vi "test timestamp from be bytes.vi"(8 "error in (no error)":errorcluster, 11 "TestCase in":refnum<class "Timestamp Tests.lvclass">) -> (0 "error out":errorcluster, 3 "TestCase out":refnum<class "Timestamp Tests.lvclass">)   [LabVIEW 2020, in "Timestamp Tests.lvclass"]
uses:
  Timestamp Tests.lvclass
  <vilib>/Utility/file.llb/Application Directory.vi
  <vilib>/Utility/libraryn.llb/Check if File or Folder Exists.vi
  <vilib>/addons/_JKI Toolkits/VI Tester/TestCase.llb/TestCase.lvclass
  C:/Program Files/National Instruments/LabVIEW 2024/vi.lib/addons/_JKI Toolkits/VI Tester/TestCase.llb/TestCase.lvclass
panel:
  out "data string":string
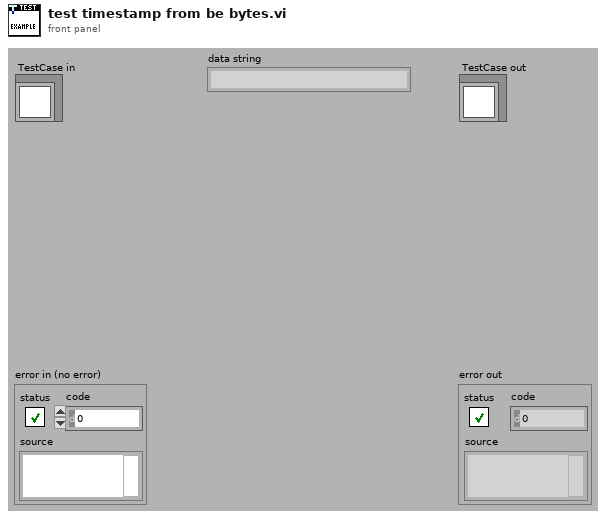
[diagram p1: front panel]
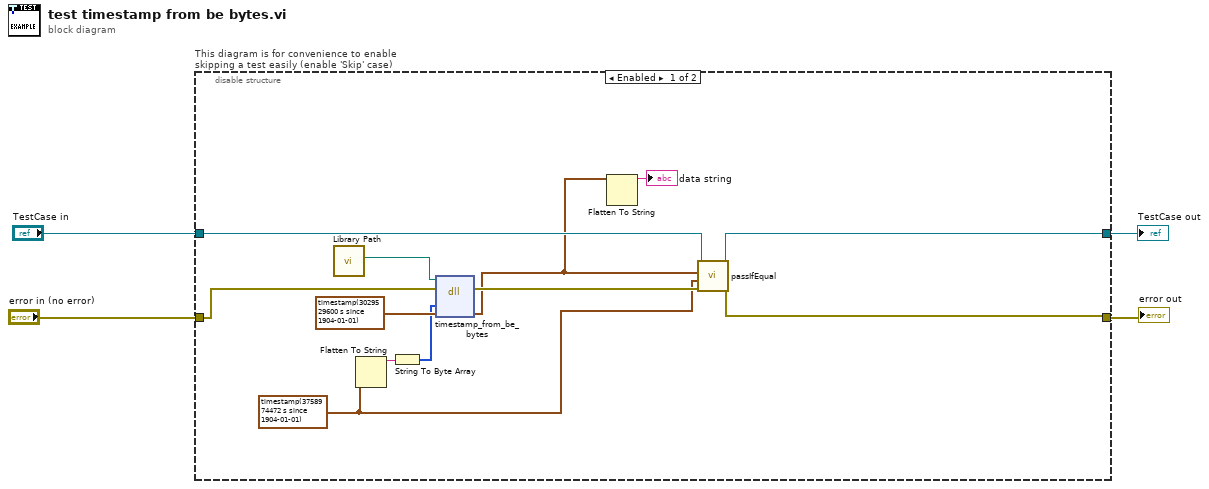
[diagram p0: block diagram]
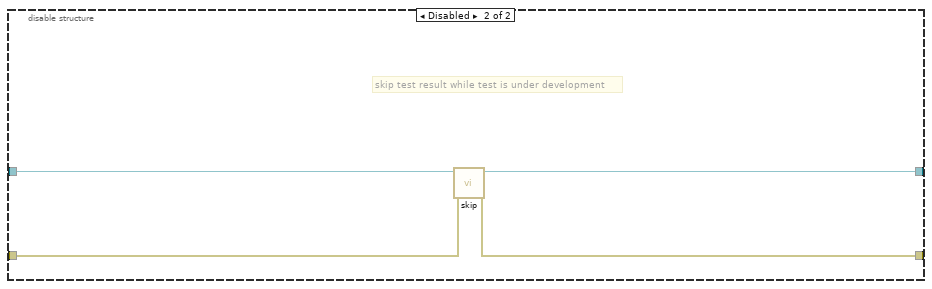
[diagram p2: hidden frame]
diagram:
  n1 = disable-structure "This diagram is for convenience to enable skipping a test easily (enable 'Skip' case)" shown="Enabled" {
    disable-tunnel: "TestCase in" -> [w16 w20]
    disable-tunnel: [w15 w18] -> w1
    disable-tunnel: [w14 w19] -> w3
    disable-tunnel: "error in (no error)" -> [w13 w17]
    frame Enabled {
      w10 = timestamp(3758974472.02441 s since 1904-01-01) ("Time Stamp")
      n2 = call "Library Path.vi"() -> ("Library Path"=w7:path)  [unwired: 11 in]
      n3 = Flatten To String(anything=w10) -> (data string=w9:string)  [unwired: 3 in, 2 out]
      n4 = String To Byte Array(string=w9) -> (unsigned byte array=w8:u8[])
      n5 = dll-call lib="C:/Users/JamesMcNally/Documents/RustInterop/Rust-LabVIEW-Interop/target/debug/labview_test_library.dll" fn="timestamp_from_be_bytes"(path in=w7, error in=w13, "bytes"=w8, "timestamp"=timestamp(3029529600 s since 1904-01-01) ("Time Stamp")) -> (error out=w12:errorcluster, "timestamp"=w6:timestamp)  [unwired: 3 in, 1 out]
      n6 = Flatten To String(anything=w6) -> (data string=→"data string":string)  [unwired: 3 in, 2 out]
      n7 = call-dynamic "passIfEqual.vi"("error in (no error)"=w12, "y"=w10, "x"=w6, "TestCase in"=w16) -> ("error out"=w14:errorcluster, "TestCase out"=w15:refnum<class "Timestamp Tests.lvclass">)  [unwired: 6 in]
    }
    frame Disabled {
      # "skip test result while test is under development"
      n8 = call <vilib>:"skip.vi"("error in (no error)"=w17, "TestCase in"=w20) -> ("error out"=w19:errorcluster, "TestCase out"=w18:refnum<class "Timestamp Tests.lvclass">)  [unwired: 8 in]
    }
  }
  "error out" <- w3
  "TestCase out" <- w1
